vi "LJstreamUD apply formula to array - no scaling.vi"(0 "Index":i32, 1 "Input Values":dbl[][](array[numeric]) format="%.2f", 2 "Variables Input":string[](array[string])=["v1", "v2", "v3", "v4"], 3 "formula":string, 4 "error in (no error)":errorcluster) -> (5 "Output Values":dbl[](array[numeric]) format="%.2f", 6 "error out":errorcluster)   [LabVIEW 2021]
doc: "Similar to the Formula Node function, but with variables that can be entered on the front panel."
panel:
  # "Input = v\nOutput = y"
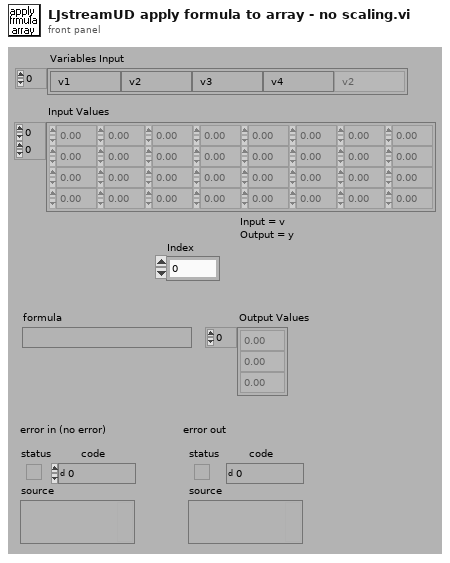
[diagram p1: front panel]
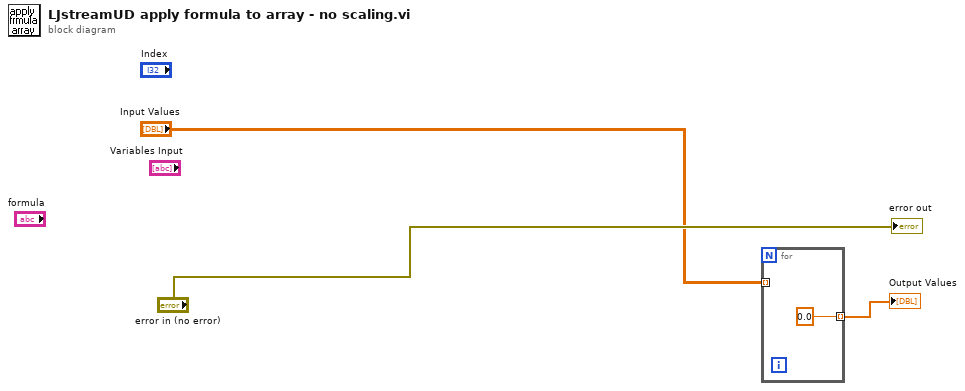
[diagram p0: block diagram]
diagram:
  n1 = for {
    tunnel: "Input Values" -> [_] mode=indexing
    tunnel: [0.0] -> w1 mode=indexing
  }
  "Output Values" <- w1
  "error out" <- "error in (no error)"
